vi "CalulateAngle.vi"(8 "D":dbl, 9 "C":dbl, 10 "B":dbl, 11 "A":dbl) -> (0 "wheelAngle4":dbl, 1 "wheelAngle3":dbl, 2 "wheelAngle2":dbl, 3 "wheelAngle1":dbl)   [LabVIEW 2019]
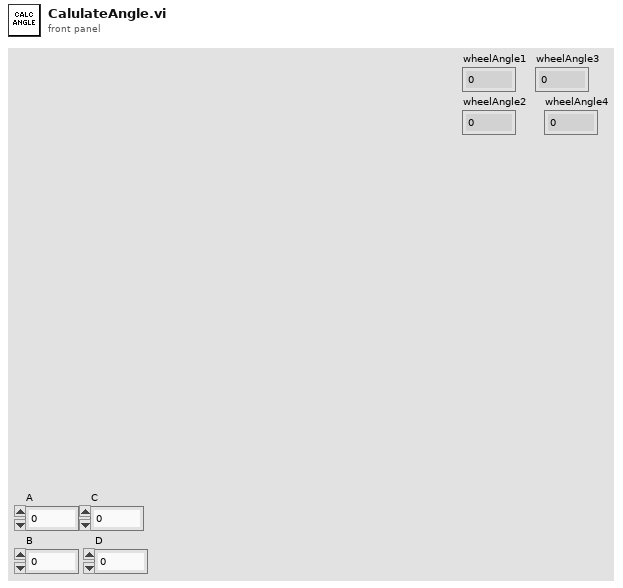
[diagram p1: front panel]
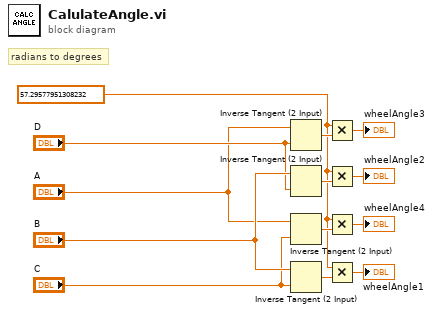
[diagram p0: block diagram]
diagram:
  w5 = 57.29577951308232 ("x")
  # "radians to degrees"
  n1 = Inverse Tangent (2 Input)(1:"D", 2:"A") -> (0:w11:dbl)
  n2 = Inverse Tangent (2 Input)(1:"D", 2:"B") -> (0:w12:dbl)
  n3 = Inverse Tangent (2 Input)(1:"C", 2:"A") -> (0:w10:dbl)
  n4 = Inverse Tangent (2 Input)(1:"C", 2:"B") -> (0:w13:dbl)
  n5 = Multiply(x=w5, y=w11) -> (x*y=→"wheelAngle3":dbl)
  n6 = Multiply(x=w5, y=w12) -> (x*y=→"wheelAngle2":dbl)
  n7 = Multiply(x=w5, y=w10) -> (x*y=→"wheelAngle4":dbl)
  n8 = Multiply(x=w5, y=w13) -> (x*y=→"wheelAngle1":dbl)
